vi "Send Multiple Messages to Notebook.vi"(6 "Error In":errorcluster, 7 "[Notebook Message]":T1[](array[typedef]) {"Message Style"."Text Alignment" items=["Left", "Right", "Center"]}, 9 "Notebook Queue":refnum<queue>) -> (0 "Error Out":errorcluster, 3 "Notebook Queue":refnum<queue>)   [LabVIEW 2021, in "Notebook.lvlib"]
doc: "This VI executes no matter what the <B>Error in</B> value is.\nThe error is passed unchanged to <B>Error out</B>, or, if there is an error when sending the message, with that new error appended to the incoming one."
uses:
  Notebook.lvlib
  Notebook Action Q Element.ctl
  Rich Text Box/Text Formatting.ctl
  Rich Text Box/Rich Text Box.lvlib
  Notebook Action List.ctl
  Rich Text Box/Text Colors.ctl
  Notebook Message Object.ctl
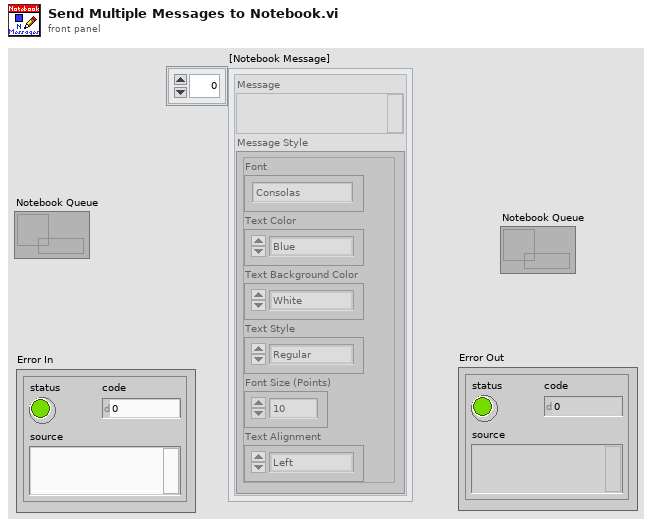
[diagram p1: front panel]
types:
  T1 = typedef "Notebook.lvlib/Notebook Message Object.ctl" = cluster{"Message":string, "Message Style":T2}
  T2 = typedef "Rich Text Box.lvlib/Text Formatting.ctl" = cluster{"Font":string, "Text Color":T3, "Text Background Color":T3, "Text Style":enum16{"Regular", "Bold", "Italic", "Underline", "Strikeout"}, "Font Size (Points)":dbl, "Text Alignment":i32}
  T3 = typedef "Rich Text Box.lvlib/Text Colors.ctl" = enum16{"Unchanged", "Black", "Blue", "Brown", "Gray", "Green", "Orange", "Pink", "Red", "White"}
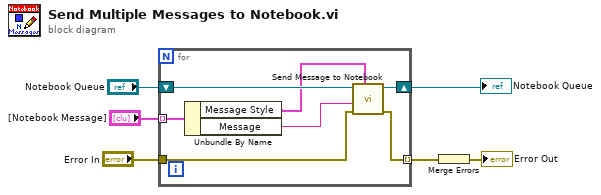
[diagram p0: block diagram]
diagram:
  n1 = for {
    shift-right: [w12] -> w4
    shift-left: "Notebook Queue" -> [w13]
    tunnel: "[Notebook Message]" -> [w9] mode=indexing
    tunnel: "Error In" -> [w11]
    tunnel: [w10] -> w2 mode=indexing
    n2 = Unbundle By Name(w9) -> ("Message Style"=w8:T2, "Message"=w7:string)
    n3 = call "Send Message to Notebook.vi"("Text Formatting"=w8, "Error In"=w11, "Message"=w7, "Notebook Queue"=w13) -> ("Error Out"=w10:errorcluster, "Notebook Queue"=w12:refnum<queue>)  [unwired: 4 in]
  }
  "Notebook Queue" <- w4
  n4 = Merge Errors(w2) -> (→"Error Out":errorcluster)
